vi "Apply Key Regular Expression.vi"(4 "Replace":string, 5 "Key name":string, 6 "Regex":string, 7 "Section name":string, 8 "error in (no error)":errorcluster, 9 "RegEx? search [T]":bool=TRUE, 10 "Replace all? [F]":bool, 11 "Carya Config in":refnum<class "Carya Config.lvclass">) -> (0 "error out":errorcluster, 3 "Carya Config out":refnum<class "Carya Config.lvclass">)   [LabVIEW 2013, in "Carya Config.lvclass"]
doc: "Copyright 2018, Carya Automatisering, Wiebe Walstra."
uses:
  Carya Config.lvclass
  CConfig Object/Search Replace Query/Search Replace Query.lvclass
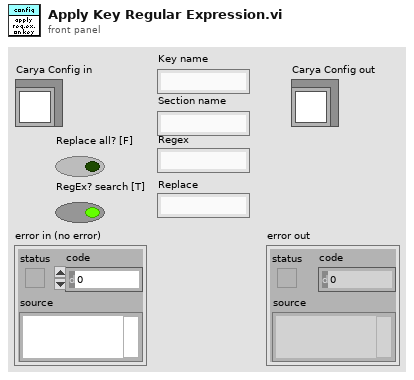
[diagram p1: front panel]
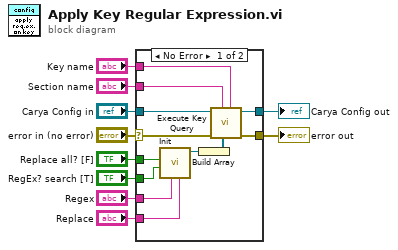
[diagram p0: block diagram]
diagram:
  n1 = case shown="No Error" "error in (no error)" {
    selector: "error in (no error)" -> [w22 w24]
    tunnel: [w21 w24] -> w9
    tunnel: [w20 w23] -> w7
    tunnel: "Carya Config in" -> [w19 w23]
    tunnel: "Section name" -> [w13 _]
    tunnel: "Key name" -> [w14 _]
    tunnel: "Regex" -> [w17 _]
    tunnel: "Replace" -> [w16 _]
    tunnel: "Replace all? [F]" -> [w18 _]
    tunnel: "RegEx? search [T]" -> [w15 _]
    frame No Error {
      n2 = call "Init.vi"("Replace"=w16, "Search"=w17, "RegEx search [T]"=w15, "Replace all? [F]"=w18) -> ("Find First Query out"=w12:refnum<class "Search Replace Query.lvclass">)  [unwired: 6 in, 1 out]
      n3 = Build Array(w12) -> (w11:refnum<class "Search Replace Query.lvclass">[])
      n4 = call-dynamic "Execute Key Query.vi"("Key name"=w14, "Key queries"=w11, "Section name"=w13, "error in (no error)"=w22, "Carya Config in"=w19) -> ("error out"=w21:errorcluster, "Carya Config out"=w20:refnum<class "Carya Config.lvclass">)  [unwired: 4 in, 1 out]
    }
    frame Error {
    }
  }
  "error out" <- w9
  "Carya Config out" <- w7
